vi "TagToFrame_Core(array)__slk_mt.vi"(7 "casemonitor in":refnum<class "CaseModel__slk_mt.lvclass">=refnum, 8 "error in (no error)":errorcluster, 11 "tags":string[](array[string])) -> (0 "error out":errorcluster, 3 "frames":string[](array[string]))   [LabVIEW 2010]
uses:
  Class/CaseModel/CaseModel__slk_mt.lvclass
  Class/DatatypeAdapter/DatatypeAdapter__slk_mt.lvclass
  Class/BooleanAdapter/BooleanAdapter__slk_mt.lvclass
  Class/NumericAdapter/NumericAdapter__slk_mt.lvclass
  Class/StringAdapter/StringAdapter__slk_mt.lvclass
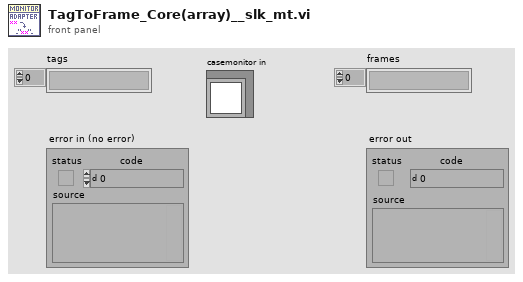
[diagram p1: front panel]
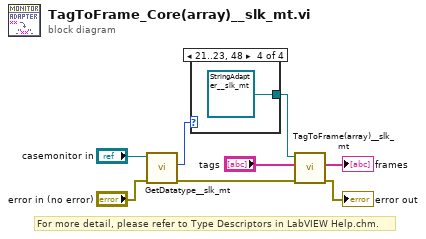
[diagram p0: block diagram]
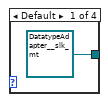
[diagram p2: hidden frame]
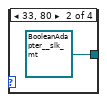
[diagram p3: hidden frame]
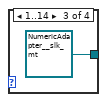
[diagram p4: hidden frame]
diagram:
  # "For more detail, please refer to Type Descriptors in LabVIEW Help.chm."
  n1 = call "GetDatatype__slk_mt.vi"("error in (no error)"="error in (no error)", "case model in"="casemonitor in") -> ("error out"=w6:errorcluster, "datatype"=w7:u8)  [unwired: 7 in, 1 out]
  n2 = case shown="21..23, 48" w7 {
    tunnel: [refnum<class "DatatypeAdapter__slk_mt.lvclass"> refnum ("CaseMonitor.lvlib:DatatypeAdapter.lvclass") refnum<class "BooleanAdapter__slk_mt.lvclass"> refnum ("CaseMonitor.lvlib:BooleanAdapter.lvclass") refnum<class "NumericAdapter__slk_mt.lvclass"> refnum ("CaseMonitor.lvlib:NumericAdapter.lvclass") refnum<class "StringAdapter__slk_mt.lvclass"> refnum ("CaseMonitor.lvlib:StringAdapter.lvclass")] -> w5
    frame Default {
    }
    frame 33, 80 {
    }
    frame 1..14 {
    }
    frame 21..23, 48 {
    }
  }
  n3 = call-dynamic "TagToFrame(array)__slk_mt.vi"("error in (no error)"=w6, "tags"="tags", "adapter in"=w5) -> ("error out"=→"error out":errorcluster, "frames"=→"frames":string[])  [unwired: 6 in, 1 out]
